vi "convert current.vi"(4 "error in":errorcluster, 7 "input string":string) -> (0 "error IO":errorcluster, 1 "remaining string":string, 2 "before substring":string, 3 "Numeric":dbl)   [LabVIEW 2018]
uses:
  <vilib>/regexp/Match Regular Expression.xnode
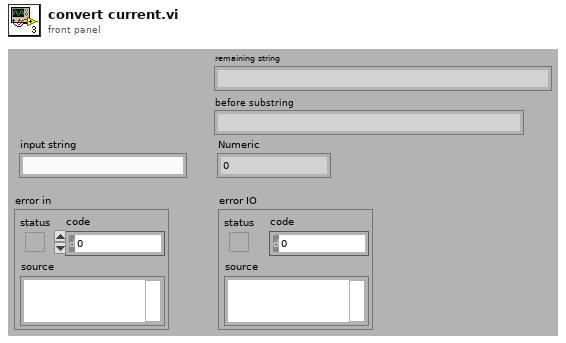
[diagram p1: front panel]
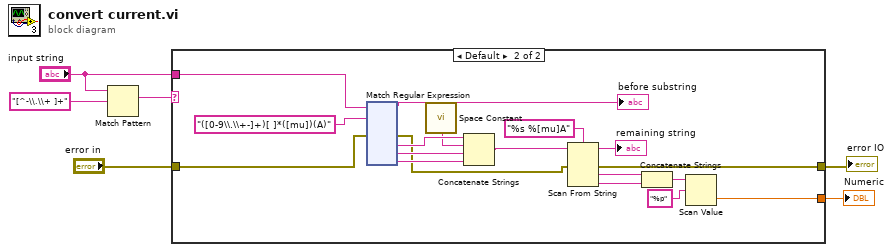
[diagram p0: block diagram]
diagram:
  n1 = Match Pattern(string="input string", regular expression="[^-\\.\\+ ]+") -> (match substring=w1:string)  [unwired: 1 in, 3 out]
  n2 = case shown="Default" w1 {
    tunnel: [w7 w20] -> w6
    tunnel: [_ w8] -> w5
    tunnel: "error in" -> [w7 w10]
    tunnel: "input string" -> [_ w9]
    frame "" {
    }
    frame Default {
      n3 = xnode "Match Regular Expression"("input string"=w9, "regular expression"="([0-9\\.\\+-]+)[ ]*([mu])(A)", "error in"=w10) -> ("before match"=→"before substring":string, "error out"=w11:errorcluster, "submatch 1"=w17:string, "submatch 2"=w15:string, "submatch 3"=w14:string)  [unwired: 3 in, 3 out]
      n4 = call <vilib>:"Space Constant.vi"() -> ("String"=w16:string)
      n5 = Concatenate Strings(w17, w16, w15, w14) -> (w13:string)
      n6 = Scan From String(format string="%s %[mu]A", input string=w13, error in=w11) -> (remaining string=→"remaining string":string, error out=w20:errorcluster, output 1=w22:string, output 2=w23:string)  [unwired: 3 in, 1 out]
      n7 = Concatenate Strings(w22, w23) -> (w24:string)
      n8 = Scan Value(string=w24, format string="%p") -> (value=w8:dbl)  [unwired: 1 in, 1 out]
    }
  }
  "Numeric" <- w5
  "error IO" <- w6
